vi "Data Message_List.vi"(7 "Parent Index":i32=-1, 8 "error in":errorcluster, 11 "SECS-II Class in":refnum<class "SECS-II Class.lvclass">) -> (0 "error out":errorcluster, 2 "Index":i32, 3 "SECS-II Class out":refnum<class "SECS-II Class.lvclass">)   [LabVIEW 2020, in "SECS Communication.lvlib" / "SECS-II Class.lvclass"]
uses:
  SECS-II Class.lvclass
  SECS-II Class.lvclass/SECS-II Class.ctl
  Format Code.ctl
  Message Data.ctl
  Data Item Format.ctl
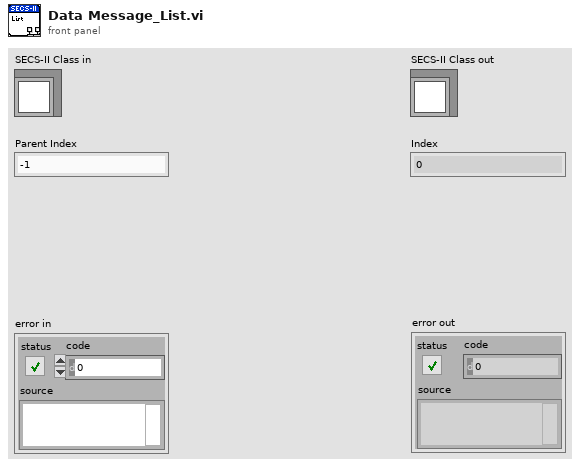
[diagram p1: front panel]
types:
  T1 = typedef "SECS Communication.lvlib/SECS-II Class.lvclass/Message Data.ctl" = cluster{"Index":i32, "Data Item Format":T2, "Format Code":T3, "Parent Index":i32, "Child Index":i32[], "Data":variant}
  T2 = typedef "SECS Communication.lvlib/SECS-II Class.lvclass/Data Item Format.ctl" = enum16{"Data Type", "Value"}
  T3 = typedef "SECS Communication.lvlib/SECS-II Class.lvclass/Format Code.ctl" = enum16{"L", "A", "B", "Boolean", "J", "I1", "I2", "I4", "I8", "U1", "U2", "U4", "U8", "F4", "F8", "Char"}
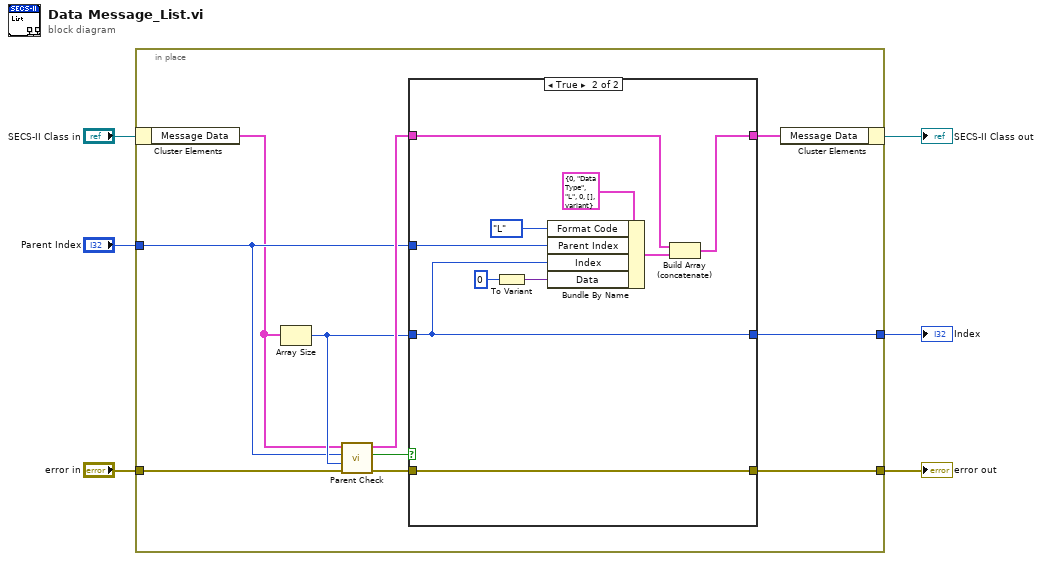
[diagram p0: block diagram]
diagram:
  n1 = in-place {
    in-place-border: "error in" -> [w16]
    in-place-border: [w11] -> w3
    in-place-border: "Parent Index" -> [w10]
    in-place-border: [w7] -> w1
    n2 = in-place-cluster #1("SECS-II Class in") -> ("Message Data"=w9:T1[])
    n3 = Array Size(array=w9) -> (size(s)=w12:i32)
    n4 = call "Parent Check.vi"("error in"=w16, "Message Index"=w12, "Parent Index"=w10, "Message Data In"=w9) -> ("error out"=w14:errorcluster, "OK?"=w15:bool, "Message Data Out"=w13:T1[])  [unwired: 5 in]
    n5 = case shown="True" w15 {
      tunnel: w14 -> [w18 w25]
      tunnel: w13 -> [w19 w27]
      tunnel: [w19 w26] -> w8
      tunnel: w10 -> [_ w28]
      tunnel: w12 -> [w17 w20]
      tunnel: [w18 w25] -> w11
      tunnel: [w17 w20] -> w7
      frame False {
      }
      frame True {
        n6 = To Variant(anything=0) -> (Variant=w22:variant)
        n7 = Bundle By Name(cluster=T1 {"Index"=0, "Data Item Format"=enum."Data Type", "Format Code"=enum."L", "Parent Index"=0, "Child Index"=[], "Data"=variant} ("Message Data"), "Format Code"=Format_Code."L", "Parent Index"=w28, "Index"=w20, "Data"=w22) -> (w21:T1)
        n8 = Build Array (concatenate)(w27, w21) -> (w26:T1[])
      }
    }
    n9 = in-place-cluster #1("Message Data"=w8) -> (→"SECS-II Class out":refnum<class "SECS-II Class.lvclass">)
  }
  "error out" <- w3
  "Index" <- w1
